vi "SendMotorCommand.vi"(8 "Command Index":dbl, 10 "Motor In":refnum<visa-resource-name>, 11 "Motor Commands":T1(array[cluster])) -> (2 "Motor Out":refnum<visa-resource-name>)   [LabVIEW 2011]
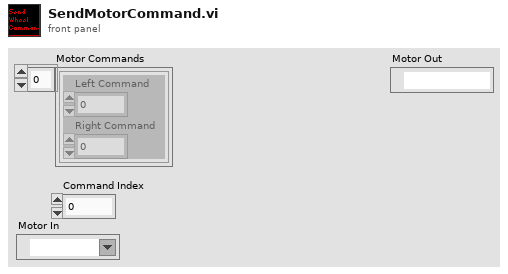
[diagram p1: front panel]
types:
  T1 = cluster{"Left Command":dbl, "Right Command":dbl}[]
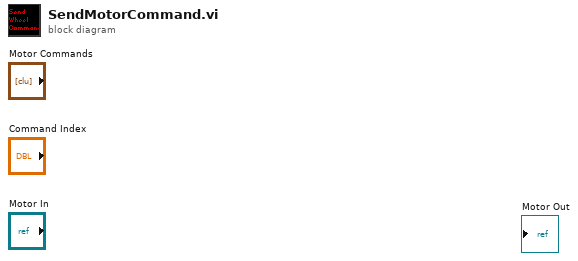
[diagram p0: block diagram]
diagram:
